vi "Add Handler.vi"(8 "error in (no error)":errorcluster, 10 "Handler":refnum<class "Handler.lvclass">, 11 "Logger in":refnum<class "Logger.lvclass">) -> (0 "error out":errorcluster, 3 "Logger out":refnum<class "Logger.lvclass">)   [LabVIEW 2017, in "Error Log.lvlib" / "Logger.lvclass"]
uses:
  Logger.lvclass
  Handler/Handler.lvclass
  Logger.lvclass/Logger.ctl
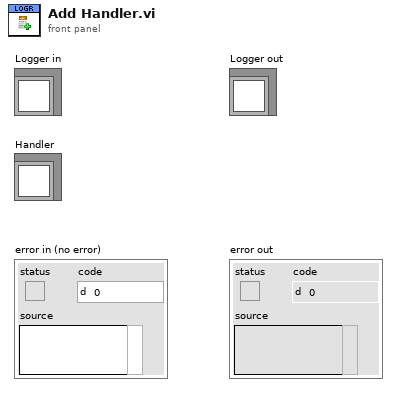
[diagram p1: front panel]
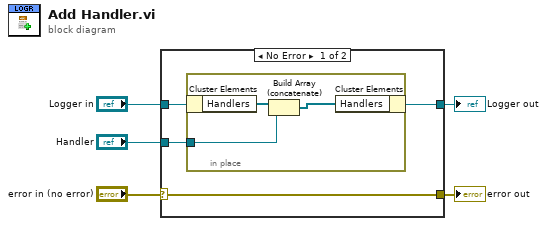
[diagram p0: block diagram]
diagram:
  n1 = case shown="No Error" "error in (no error)" {
    selector: "error in (no error)" -> [w8 w14]
    tunnel: [w8 w14] -> w4
    tunnel: [w9 w13] -> w2
    tunnel: "Logger in" -> [w7 w13]
    tunnel: "Handler" -> [w6 _]
    frame No Error {
      n2 = in-place {
        in-place-border: w6 -> [w10]
        n3 = in-place-cluster #1(w7) -> ("Handlers"=w12:refnum<class "Handler.lvclass">[])
        n4 = Build Array (concatenate)(w12, w10) -> (w11:refnum<class "Handler.lvclass">[])
        n5 = in-place-cluster #1("Handlers"=w11) -> (w9:refnum<class "Logger.lvclass">)
      }
    }
    frame Error {
    }
  }
  "error out" <- w4
  "Logger out" <- w2
